vi "Custom Warning.vi"() -> ()   [LabVIEW 2013]
uses:
  <vilib>/Utility/error.llb/DialogType.ctl
panel:
  out "error out":errorcluster
  in  "error in (no error)":errorcluster={"status"=FALSE, "code"=5000, "source"=""}
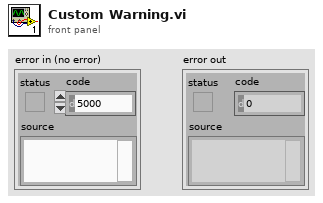
[diagram p1: front panel]
types:
  T1 = typedef "DialogType.ctl" = u16
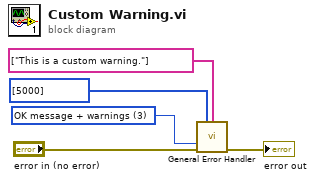
[diagram p0: block diagram]
diagram:
  w5 = T1 3 items=["no dialog", "OK message", "continue or stop message", "OK message + warnings", "continue/stop + warnings"] ("type of dialog (OK msg:1)")
  n1 = call <vilib>:"General Error Handler.vi"("[user-defined codes]"=i32[] [5000], "[user-defined descriptions]"=string[] ["This is a custom warning."], "type of dialog (OK msg:1)"=w5, "error in (no error)"="error in (no error)") -> ("error out"=→"error out":errorcluster)  [unwired: 7 in, 4 out]
